vi "Load or create a para cfg.vi"(8 "error in":errorcluster, 10 "Tree Refnum":refnum<vi>, 11 "Tbl Refnum in":refnum<vi>) -> (0 "error out":errorcluster, 1 "cfg file refnum out":refnum<file>, 2 "Tree Refnum out":refnum<vi>, 3 "Tbl Refnum out":refnum<vi>)   [LabVIEW 2010]
uses:
  <vilib>/Utility/miscctls.llb/LVRowAndColumnTypeDef.ctl
panel:
  out "All Tags":string[](array[string])
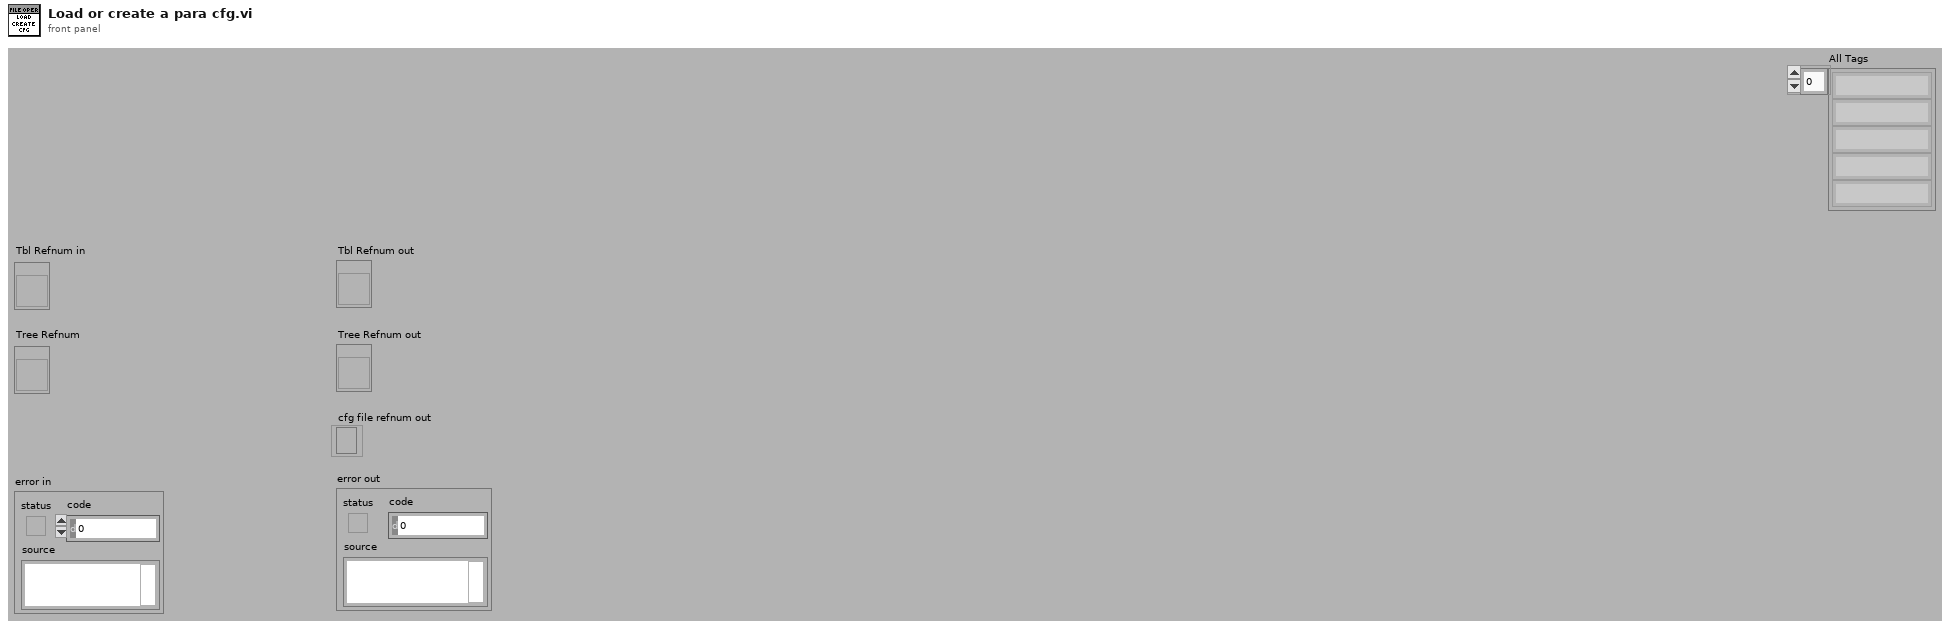
[diagram p1: front panel]
types:
  T1 = typedef "LVRowAndColumnTypeDef.ctl" = cluster{"Row":i32, "Column":i32}
  T2 = enum16{"open", "replace", "create", "open or create", "replace or create", "replace or create with confirmation"}
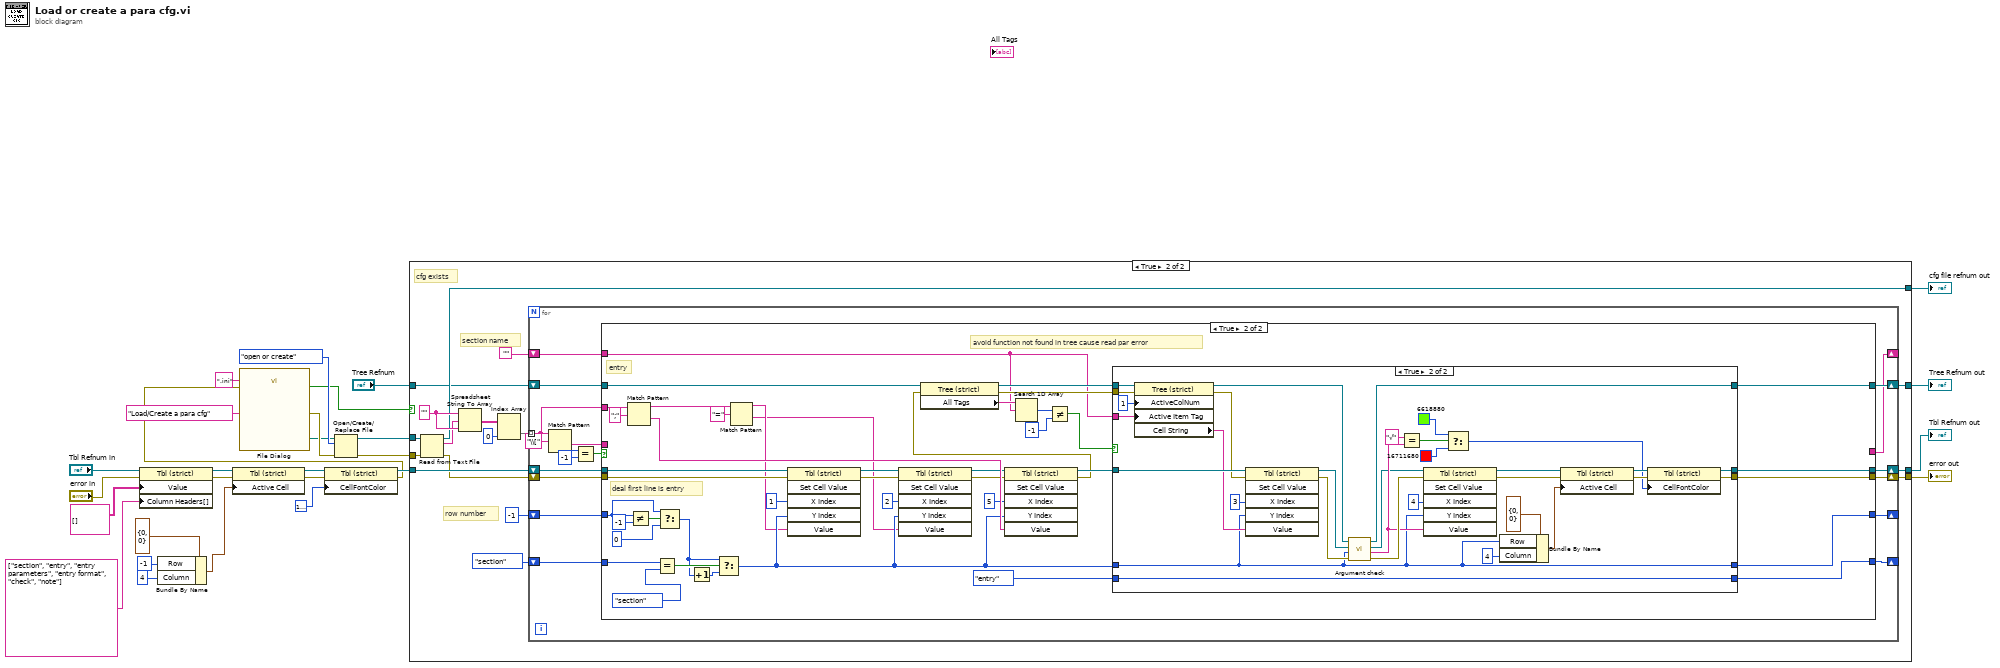
[diagram p0: block diagram]
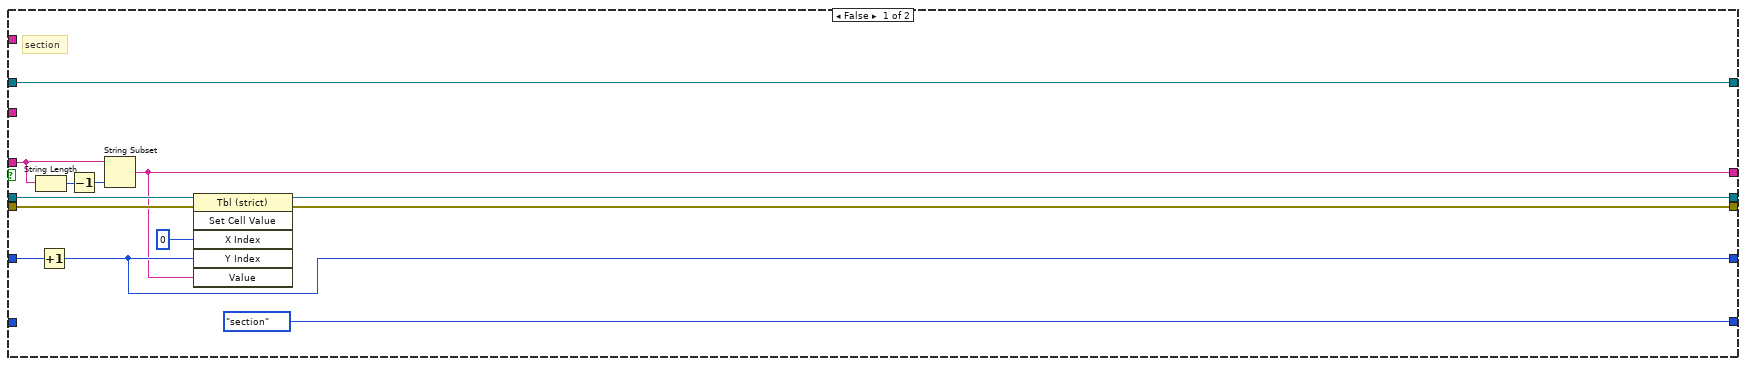
[diagram p3: hidden frame]
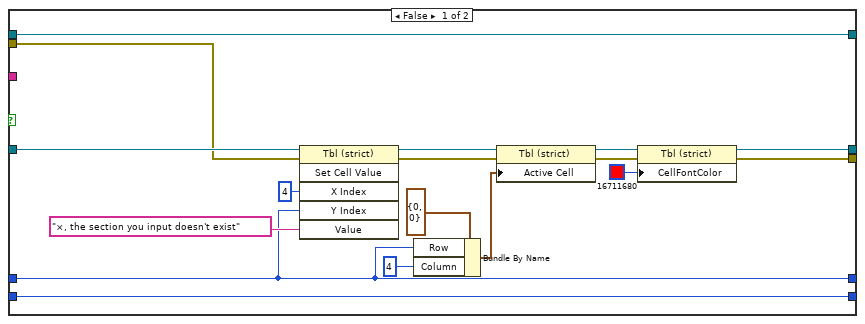
[diagram p4: hidden frame]
diagram:
  n1 = property class="Tbl (strict)"(reference="Tbl Refnum in", error in="error in", "Value"=string[][] [], "Column Headers[]"=string[] ["section", "entry", "entry parameters", "entry format", "check", "note"] ("Row Header Strings[]")) -> (reference out=w11:refnum<vi>, error out=w10:errorcluster)
  n2 = Bundle By Name(cluster=T1 {"Row"=0, "Column"=0} ("Active Cell:Active Cell"), "Row"=-1, "Column"=4) -> (w6:T1)
  n3 = property on="Property Node" class="Tbl (strict)"(reference=w11, error in=w10, "Active Cell"=w6) -> (reference out=w5:refnum<vi>, error out=w4:errorcluster)
  n4 = property on="Property Node" class="Tbl (strict)"(reference=w5, error in=w4, "CellFontColor"=u32 16777222) -> (reference out=w3:refnum<vi>, error out=w2:errorcluster)
  n5 = call "File Dialog"("prompt"="Load/Create a para cfg", "default name"=".ini", "error in"=w2) -> ("selected path"=w26:path, "exists"=w25:bool, "error out"=w27:errorcluster)  [unwired: 9 in, 1 out]
  n6 = Open/Create/Replace File(file path (use dialog)=w26, error in=w27, operation (0:open)=T2."open or create") -> (refnum out=w24:refnum<file>, error out=w23:errorcluster)  [unwired: 3 in, 1 out]
  n7 = case shown="True" w25 {
    tunnel: w24 -> [w32 w45]
    tunnel: w23 -> [w31 w44]
    tunnel: w3 -> [w30 w42]
    tunnel: [w32 w39] -> w17
    tunnel: [w31 w38] -> w16
    tunnel: [w30 w36] -> w15
    tunnel: "Tree Refnum" -> [w29 w35]
    tunnel: [w29 w34] -> w13
    frame False {
      # "create a new cfg"
    }
    frame True {
      w47 = ""
      # "section name"
      # "row number"
      # "cfg exists"
      n8 = Read from Text File(file (use dialog)=w45, error in=w44) -> (refnum out=w39:refnum<file>, text=w46:string, error out=w37:errorcluster)  [unwired: 2 in, 1 out]
      n9 = Spreadsheet String To Array(format string=w47, spreadsheet string=w46, array type (2D Dbl)=w47) -> (array=w48:string[][])  [unwired: 1 in]
      n10 = Index Array(array=w48, index (col)=0 ("disabled index (col)")) -> (element=w43:string[])  [unwired: 1 in]
      n11 = for {
        tunnel: w43 -> [w61] mode=indexing
        shift-right: [w59] -> _
        shift-left: -1 -> [w63]
        shift-right: [w58] -> _
        shift-left: enum16{"section", "entry"}."section" -> [w57]
        shift-right: [w56] -> w38
        shift-left: w37 -> [w55]
        shift-right: [w54] -> w36
        shift-left: w42 -> [w60]
        shift-right: [w52] -> w34
        shift-left: w35 -> [w53]
        shift-right: [w51] -> _
        shift-left: "" -> [w50]
        n12 = Match Pattern(string=w61, regular expression="\\[") -> (after substring=w62:string, offset past match=w66:i32)  [unwired: 1 in, 2 out]
        n13 = Equal?(x=w66, y=-1) -> (x = y?=w64:bool)
        n14 = case shown="True" w64 {
          tunnel: w63 -> [w75 w121]
          tunnel: [w74 w120] -> w59
          tunnel: w62 -> [w80 _]
          tunnel: w61 -> [_ w114]
          tunnel: w60 -> [w77 w122]
          tunnel: [enum16{"section", "entry"}."section" w119] -> w58
          tunnel: w57 -> [_ w118]
          tunnel: w55 -> [w72 w117]
          tunnel: [w71 w116] -> w56
          tunnel: [w70 w115] -> w54
          tunnel: w53 -> [w69 w111]
          tunnel: [w69 w110] -> w52
          tunnel: [w68 _] -> w51
          tunnel: w50 -> [_ w81]
          frame False {
            # "section"
            n15 = String Length(string=w80) -> (length=w79:i32)
            n16 = Increment(x=w75) -> (x+1=w74:i32)
            n17 = Decrement(x=w79) -> (x-1=w78:i32)
            n18 = String Subset(string=w80, length (rest)=w78) -> (substring=w68:string)  [unwired: 1 in]
            n19 = invoke class="Tbl (strict)" method="Set Cell Value"(reference=w77, error in=w72, "X Index"=u32 0 ("Y Index"), "Y Index"=w74, "Value"=w68) -> (reference out=w70:refnum<vi>, error out=w71:errorcluster)  [unwired: 1 in, 4 out]
          }
          frame True {
            # "avoid function not found in tree cause read par error"
            # "deal first line is entry"
            # "entry"
            n20 = Match Pattern(string=w114, regular expression=";") -> (before substring=w112:string, after substring=w109:string)  [unwired: 1 in, 2 out]
            n21 = Not Equal?(x=w121, y=-1) -> (x != y?=w92:bool)
            n22 = Equal?(x=w118, y=enum16{"section", "entry"}."section") -> (x = y?=w106:bool)
            n23 = Select(t=w121, s=w92, f=0) -> (s? t:f=w90:i32)
            n24 = Increment(x=w90) -> (x+1=w105:i32)
            n25 = Select(t=w90, s=w106, f=w105) -> (s? t:f=w86:i32)
            n26 = Match Pattern(string=w112, regular expression="=") -> (before substring=w83:string, after substring=w82:string)  [unwired: 1 in, 2 out]
            n27 = invoke class="Tbl (strict)" method="Set Cell Value"(reference=w122, error in=w117, "X Index"=u32 1, "Y Index"=w86, "Value"=w83) -> (reference out=w102:refnum<vi>, error out=w103:errorcluster)  [unwired: 1 in, 4 out]
            n28 = invoke class="Tbl (strict)" method="Set Cell Value"(reference=w102, error in=w103, "X Index"=u32 2, "Y Index"=w86, "Value"=w82) -> (reference out=w89:refnum<vi>, error out=w88:errorcluster)  [unwired: 1 in, 4 out]
            n29 = invoke class="Tbl (strict)" method="Set Cell Value"(reference=w89, error in=w88, "X Index"=u32 5, "Y Index"=w86, "Value"=w109) -> (reference out=w85:refnum<vi>, error out=w84:errorcluster)  [unwired: 1 in, 4 out]
            n30 = property on="Property Node" class="Tree (strict)"(reference=w111, error in=w84) -> (reference out=w98:refnum<vi>, error out=w94:errorcluster, "All Tags"=w99:string[])
            n31 = Search 1D Array(1D array=w99, element=w81) -> (index of element=w97:i32)  [unwired: 1 in]
            n32 = Not Equal?(x=w97, y=-1) -> (x != y?=w95:bool)
            n33 = case shown="True" w95 {
              tunnel: w85 -> [w137 w171]
              tunnel: [w131 w141] -> w110
              tunnel: w98 -> [w131 w167]
              tunnel: w94 -> [w136 w166]
              tunnel: w81 -> [_ w165]
              tunnel: [w124 w147] -> w115
              tunnel: [w123 w148] -> w116
              tunnel: w86 -> [w126 w140]
              tunnel: enum16{"section", "entry"}."entry" -> [w130 w160]
              tunnel: [w130 w160] -> w119
              tunnel: [w126 w140] -> w120
              frame False {
                n34 = invoke class="Tbl (strict)" method="Set Cell Value"(reference=w137, error in=w136, "X Index"=u32 4, "Y Index"=w126, "Value"="×, the section you input doesn't exist") -> (reference out=w135:refnum<vi>, error out=w134:errorcluster)  [unwired: 1 in, 4 out]
                n35 = Bundle By Name(cluster=T1 {"Row"=0, "Column"=0} ("Active Cell:Active Cell"), "Row"=w126, "Column"=4) -> (w129:T1)
                n36 = property on="Property Node" class="Tbl (strict)"(reference=w135, error in=w134, "Active Cell"=w129) -> (reference out=w128:refnum<vi>, error out=w127:errorcluster)
                n37 = property on="Property Node" class="Tbl (strict)"(reference=w128, error in=w127, "CellFontColor"=u32 16711680) -> (reference out=w124:refnum<vi>, error out=w123:errorcluster)
              }
              frame True {
                n38 = property class="Tree (strict)"(reference=w167, error in=w166, "ActiveColNum"=1 ("Active Cell:Active Column Number"), "Active Item Tag"=w165) -> (reference out=w145:refnum<vi>, error out=w168:errorcluster, "Cell String"=w161:string)
                n39 = invoke class="Tbl (strict)" method="Set Cell Value"(reference=w171, error in=w168, "X Index"=u32 3, "Y Index"=w140, "Value"=w161) -> (reference out=w143:refnum<vi>, error out=w163:errorcluster)  [unwired: 1 in, 4 out]
                n40 = call "Argument check.vi"("error in"=w163, "Row number"=w140, "Tbl Refnum in"=w143, "Tree Refnum in"=w145) -> ("error out"=w162:errorcluster, "Check result"=w144:string, "Tbl Refnum out"=w142:refnum<vi>, "Tree Refnum out"=w141:refnum<vi>)  [unwired: 4 in]
                n41 = Equal?(x="√", y=w144) -> (x = y?=w154:bool)
                n42 = invoke class="Tbl (strict)" method="Set Cell Value"(reference=w142, error in=w162, "X Index"=u32 4, "Y Index"=w140, "Value"=w144) -> (reference out=w159:refnum<vi>, error out=w158:errorcluster)  [unwired: 1 in, 4 out]
                n43 = Select(t=u32 6618880, s=w154, f=u32 16711680) -> (s? t:f=w146:u32)
                n44 = Bundle By Name(cluster=T1 {"Row"=0, "Column"=0} ("Active Cell:Active Cell"), "Row"=w140, "Column"=4) -> (w151:T1)
                n45 = property on="Property Node" class="Tbl (strict)"(reference=w159, error in=w158, "Active Cell"=w151) -> (reference out=w150:refnum<vi>, error out=w149:errorcluster)
                n46 = property on="Property Node" class="Tbl (strict)"(reference=w150, error in=w149, "CellFontColor"=w146) -> (reference out=w147:refnum<vi>, error out=w148:errorcluster)
              }
            }
          }
        }
      }
    }
  }
  "error out" <- w16
  "cfg file refnum out" <- w17
  "Tbl Refnum out" <- w15
  "Tree Refnum out" <- w13
